vi "AOGen.vi"(8 "错误输入":errorcluster caption="错误输入（无错误）", 11 "GUIRef":T1={"StringOut"=refnum, "AbortOnFail"=refnum, "SN"=refnum, "SN_Length"=refnum, "TestResult"=refnum, "CycleTime"=refnum, "ErrorCode"=refnum, "UUTStatus"=refnum, "DataBaseEnable?"=refnum, "DUTModel"=refnum, "FixtureID"=refnum, "OperatorID"=refnum, "SNReady"=refnum, "StopSlot"=refnum, "NextStep"=refnum, "PassYeild"=refnum, "Failed"=refnum, "Passed"=refnum, "Tested"=refnum, "TestItemsCtl"={"StepName"="", "TestEnable"=FALSE, "LoopCount"=0, "StopOnFail"=FALSE, "Index"=0, "TestName"="", "通道"="", "参数"="", "TimeStart"=0}, "ProcessBar"=refnum, "Slot"=enum."Slot1", "Row"=3, "States"=refnum, "TestMode"=refnum, "循环次数-DUT"=refnum, "波形图"=refnum, "产品型号"=refnum, "子面板"=refnum, "测试失败项目"=refnum, "测试结果"=refnum, "DUT"=refnum, "Starttime"=refnum, "SlotReady"=refnum, "版本信息"=refnum}) -> (0 "错误输出":errorcluster)   [LabVIEW 2013]
uses:
  SystemCode/SysControl/Reference.ctl
  SystemCode/SysControl/TestItemsCTL.ctl
  SystemCode/SysControl/Slot.ctl
  <vilib>/DAQmx/write.llb/DAQmx Write (Analog 1D Wfm NChan NSamp).vi
  GlobalValue.vi
  <vilib>/DAQmx/create/channels.llb/DAQmx Create Channel (AO-Voltage-Basic).vi
  <vilib>/DAQmx/configure/timing.llb/DAQmx Timing (Sample Clock).vi
  <vilib>/DAQmx/miscellaneous.llb/DAQmx Fill In Error Info.vi
  <resource>/objmgr/daqmx.rc
  <vilib>/measure/NI_MABase.lvlib
panel:
  in  "CH":string="MIC"
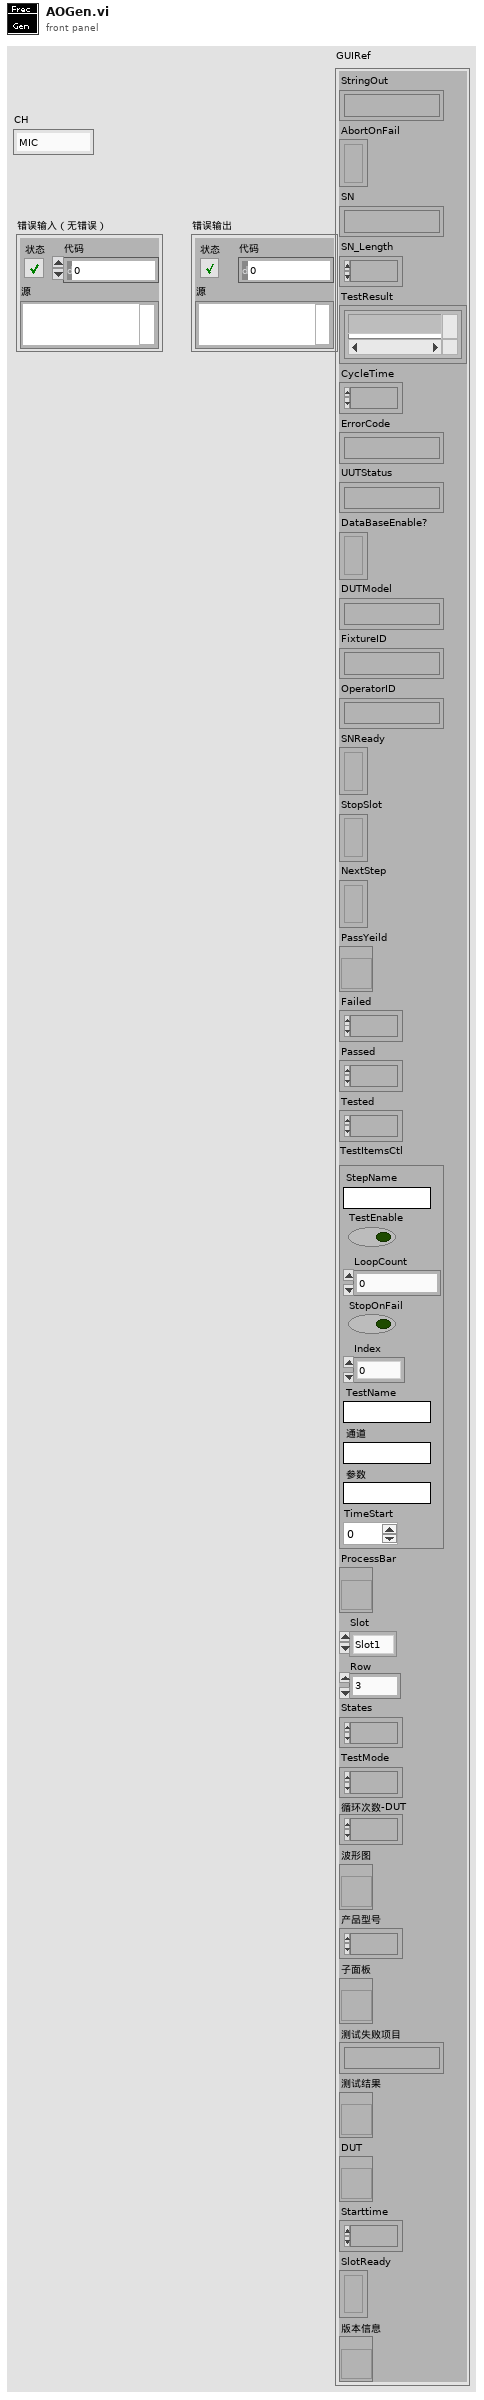
[diagram p1: front panel]
types:
  T1 = typedef "Reference.ctl" = cluster{"StringOut":refnum<vi>, "AbortOnFail":refnum<vi>, "SN":refnum<vi>, "SN_Length":refnum<vi>, "TestResult":refnum<vi>, "CycleTime":refnum<vi>, "ErrorCode":refnum<vi>, "UUTStatus":refnum<vi>, "DataBaseEnable?":refnum<vi>, "DUTModel":refnum<vi>, "FixtureID":refnum<vi>, "OperatorID":refnum<vi>, "SNReady":refnum<vi>, "StopSlot":refnum<vi>, "NextStep":refnum<vi>, "PassYeild":refnum<vi>, "Failed":refnum<vi>, "Passed":refnum<vi>, "Tested":refnum<vi>, "TestItemsCtl":T2, "ProcessBar":refnum<vi>, "Slot":T3, "Row":u32, "States":refnum<vi>, "TestMode":refnum<vi>, "循环次数-DUT":refnum<vi>, "波形图":refnum<vi>, "产品型号":refnum<vi>, "子面板":refnum<vi>, "测试失败项目":refnum<vi>, "测试结果":refnum<vi>, "DUT":refnum<vi>, "Starttime":refnum<vi>, "SlotReady":refnum<vi>, "版本信息":refnum<vi>}
  T2 = typedef "TestItemsCTL.ctl" = cluster{"StepName":string, "TestEnable":bool, "LoopCount":i32, "StopOnFail":bool, "Index":u32, "TestName":string, "通道":string, "参数":string, "TimeStart":u32}
  T3 = typedef "Slot.ctl" = enum16{"Slot1", "Slot2", "Slot3", "Slot4"}
  T4 = typedef "DAQConfig.ctl" = cluster{"DIO":string[][], "AO":string[][], "AI":string[][]}
  T5 = enum16{"Production Mode", "Selection Mode", "Debug Mode", "Loop Mode", "Stop Test"}
  T6 = enum16{"Sine Wave", "Triangle Wave", "Square Wave", "Sawtooth Wave"}
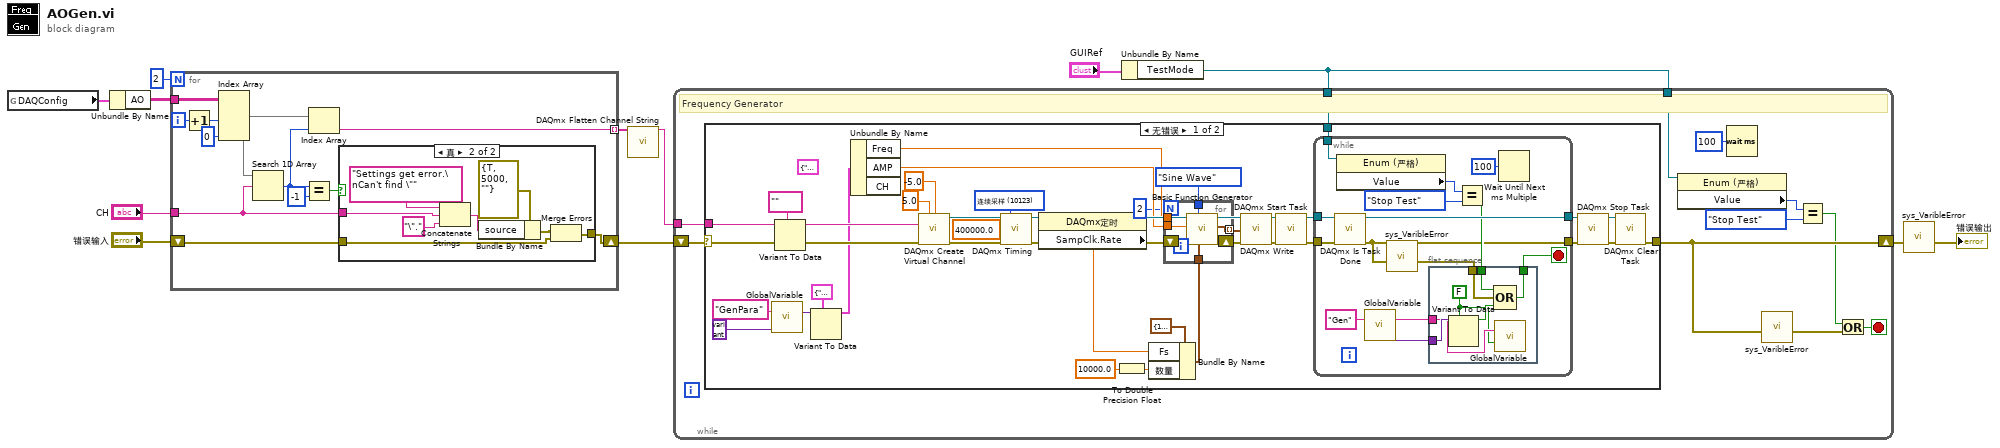
[diagram p0: block diagram]
diagram:
  n1 = global read "GlobalValue.vi" "DAQConfig"() -> (w7:T4)
  n2 = Unbundle By Name(w7) -> ("AO"=w9:string[][])
  n3 = for {
    N: 2 -> [_]
    tunnel: w9 -> [w25]
    tunnel: "CH" -> [w18]
    tunnel: [w15] -> w3 mode=indexing
    shift-right: [w17] -> w5
    shift-left: "错误输入" -> [w16]
    i -> [w14]
    n4 = Increment(x=w14) -> (x+1=w13:i32)
    n5 = Index Array(array=w25, index (col) #1=w13, index (col) #2=0 ("索引 (列)")) -> (element #1=w21:string[], element #2=w20:string[])  [unwired: 2 in]
    n6 = Search 1D Array(1D array=w20, element=w18) -> (index of element=w23:i32)  [unwired: 1 in]
    n7 = Equal?(x=w23, y=-1) -> (x = y?=w19:bool)
    n8 = Index Array(array=w21, index=w23) -> (element=w15:string)
    n9 = case shown="真" w19 {
      tunnel: w16 -> [w26 w30]
      tunnel: [w26 w29] -> w17
      tunnel: w18 -> [_ w28]
      frame False {
      }
      frame True {
        n10 = Concatenate Strings("Settings get error.\nCan't find \"" ("message"), w28, "\"." ("string")) -> (w33:string)
        n11 = Bundle By Name(cluster=errorcluster {"status"=TRUE, "code"=5000, "source"=""} ("error in 1 (no error)"), "source"=w33) -> (w32:errorcluster)
        n12 = Merge Errors(w32, w30) -> (w29:errorcluster)
      }
    }
  }
  n13 = call <vilib>:"DAQmx Flatten Channel String.vi"("names in"=w3) -> ("names out"=w2:string)  [unwired: 13 in, 1 out]
  n14 = Unbundle By Name("GUIRef") -> ("TestMode"=w1:refnum<vi>)
  n15 = while "While循环" {
    shift-right: [w43] -> w12
    shift-left: w5 -> [w44]
    tunnel: w1 -> [w42]
    tunnel: w2 -> [w37]
    tunnel: w1 -> [w36]
    stop <- w38 stop-if-true
    # "Frequency Generator"
    n16 = case shown="无错误" w44 {
      selector: w44 -> [w84 w113]
      tunnel: [w85 w113] -> w43
      tunnel: w37 -> [w83 _]
      tunnel: w36 -> [w82 _]
      frame No Error {
        (unwired) cluster{"CH":tag, "Freq":dbl, "AMP":dbl} {"CH"="PCI-6229/ai1", "Freq"=1000.0, "AMP"=0.2} ("Paras 2")
        w76 = 10123 items=["有限采样"=10178, "连续采样"=10123, "硬件定时单点"=12522] ("sample mode")
        n17 = call "GlobalVariable.vi"("Name"="GenPara", "ValueIn"=variant) -> ("ValueOut"=w48:variant)  [unwired: 10 in, 3 out]
        n18 = Variant To Data(type=tag "" ("lines"), Variant=w83) -> (data=w53:tag)  [unwired: 1 in, 1 out]
        n19 = Variant To Data(type=cluster{"CH":tag, "Freq":dbl, "AMP":dbl} {"CH"="Dev1/ao1", "Freq"=1000.0, "AMP"=0.2} ("Paras 2"), Variant=w48) -> (data=w47:cluster{"CH":tag, "Freq":dbl, "AMP":dbl})  [unwired: 1 in, 1 out]
        n20 = Unbundle By Name(w47) -> ("Freq"=w56:dbl, "AMP"=w55:dbl)  [unwired: 1 out]
        n21 = call-poly <vilib>:"DAQmx Create Virtual Channel.vi"("maximum value"=5.0, "minimum value"=-5.0, "physical channels"=w53, "error in"=w84) -> ("task out"=w79:refnum<k21>, "error out"=w78:errorcluster)  [unwired: 10 in]
        n22 = call-poly <vilib>:"DAQmx Timing.vi"("task/channels in"=w79, "sample mode"=w76, "rate"=400000.0, "error in"=w78) -> ("task out"=w75:refnum<k21>, "error out"=w71:errorcluster)  [unwired: 10 in]
        n23 = property class="DAQmx定时"(reference=w75, error in=w71) -> (reference out=w69:refnum<k21>, error out=w72:errorcluster, "SampClk.Rate"=w58:dbl)
        n24 = To Double Precision Float(number=10000.0 ("数字")) -> (double precision float=w59:dbl)
        n25 = Bundle By Name(cluster=cluster{"Fs":dbl, "数量":dbl} {"Fs"=1000.0, "数量"=1000.0} ("采样信息"), "Fs"=w58, "数量"=w59) -> (w66:cluster{"Fs":dbl, "数量":dbl})
        n26 = for {
          N: 2 -> [_]
          tunnel: T6."Sine Wave" ("signal type") -> [w91]
          tunnel: w66 -> [w90]
          tunnel: w56 -> [w88]
          tunnel: w55 -> [w87]
          shift-right: [w89] -> w65
          shift-left: w72 -> [w92]
          tunnel: [w86] -> w52 mode=indexing
          n27 = call <vilib>:"Basic Function Generator.vi"("sampling info"=w90, "signal type"=w91, "error in (no error)"=w92, "amplitude"=w87, "frequency"=w88) -> ("error out"=w89:errorcluster, "signal out"=w86:waveform(dbl))  [unwired: 4 in, 1 out]
        }
        n28 = call-poly <vilib>:"DAQmx Write.vi"("task/channels in"=w69, "data"=w52, "error in"=w65) -> ("task out"=w68:refnum<k21>, "error out"=w67:errorcluster)  [unwired: 10 in, 1 out]
        n29 = call <vilib>:"DAQmx Start Task.vi"("task/channels in"=w68, "error in"=w67) -> ("task out"=w64:refnum<k21>, "error out"=w57:errorcluster)  [unwired: 12 in]
        n30 = while {
          tunnel: w64 -> [w103]
          tunnel: w57 -> [w102]
          tunnel: [w95] -> w62
          tunnel: [w104] -> w61
          tunnel: w82 -> [w99]
          stop <- w96 stop-if-true
          w93 = "Gen" ("Name")
          n31 = call <vilib>:"DAQmx Is Task Done.vi"("task/channels in"=w103, "error in"=w102) -> ("task out"=w104:refnum<k21>, "error out"=w95:errorcluster)  [unwired: 11 in, 1 out]
          n32 = property class="Enum (严格)"(reference=w99) -> ("Value"=w100:T5)  [unwired: 1 in, 2 out]
          n33 = call "GlobalVariable.vi"("Name"=w93) -> ("ValueOut"=w94:variant)  [unwired: 11 in, 3 out]
          n34 = call "sys_VaribleError.vi"("ErrorIn"=w95) -> ("ErrorOut"=w97:errorcluster)  [unwired: 10 in]
          n35 = flat-sequence {
            tunnel: w98 -> [w112]
            tunnel: w97 -> [w111]
            tunnel: [w110] -> w96
            tunnel: w94 -> [w109]
            tunnel: w93 -> [w107]
            frame #0 {
              w106 = FALSE
              n36 = Variant To Data(type=w106, Variant=w109) -> (data=w108:bool)  [unwired: 1 in, 1 out]
              n37 = Compound Arithmetic op=OR(w112, w111, w108) -> (w110:bool)
              n38 = call "GlobalVariable.vi"("Name"=w107, "ValueIn"=w106) -> ()  [unwired: 10 in, 4 out]
            }
          }
          n39 = Equal?(x=w100, y=T5."Stop Test") -> (x = y?=w98:bool)
          n40 = Wait Until Next ms Multiple(millisecond multiple=u32 100 ("毫秒倍数")) -> ()  [unwired: 1 out]
        }
        n41 = call <vilib>:"DAQmx Stop Task.vi"("task/channels in"=w61, "error in"=w62) -> ("task out"=w60:refnum<k21>, "error out"=w63:errorcluster)  [unwired: 12 in]
        n42 = call <vilib>:"DAQmx Clear Task.vi"("task in"=w60, "error in"=w63) -> ("error out"=w85:errorcluster)  [unwired: 13 in]
      }
      frame Error {
      }
    }
    n43 = property class="Enum (严格)"(reference=w42) -> ("Value"=w41:T5)  [unwired: 1 in, 2 out]
    n44 = Wait (ms)(milliseconds to wait=u32 100 ("等待时间（毫秒）")) -> ()  [unwired: 1 out]
    n45 = call "sys_VaribleError.vi"("ErrorIn"=w43) -> ("ErrorOut"=w35:errorcluster)  [unwired: 10 in]
    n46 = Equal?(x=w41, y=T5."Stop Test") -> (x = y?=w39:bool)
    n47 = Or(x=w39, y=w35) -> (x .or. y?=w38:bool)
  }
  n48 = call "sys_VaribleError.vi"("ErrorIn"=w12) -> ("ErrorOut"=→"错误输出":errorcluster)  [unwired: 10 in]
